vi "Main Simulation Area.vi"   [LabVIEW 2013]
uses:
  <vilib>/rvi/DesktopExecutionNode/DesktopExecutionNode.xnode
  <vilib>/rvi/DesktopExecutionNode/Execution/niFpgaDEN_Execute.vi
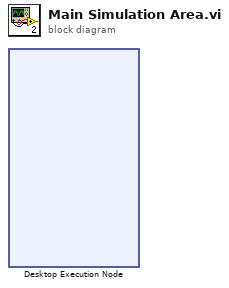
[diagram p0: block diagram]
diagram:
  n1 = xnode "Desktop Execution Node"() -> ()  [unwired: 8 in, 2 out]
